vi "Remote Set Control Value.vi"(6 "Field name":string, 8 "error in (no error)":errorcluster, 10 "Name":string, 11 "Template Module in":refnum<class "Template Module.lvclass">) -> (0 "error out":errorcluster, 3 "Template Module out":refnum<class "Template Module.lvclass">, 9 "Value":variant)   [LabVIEW 2016]
uses:
  Template Module.lvclass
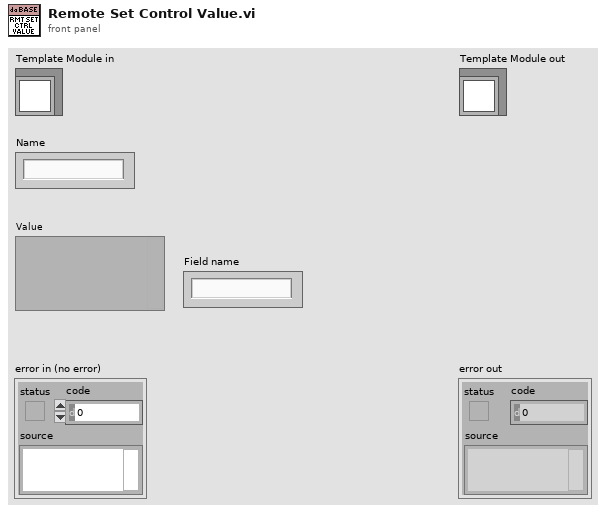
[diagram p1: front panel]
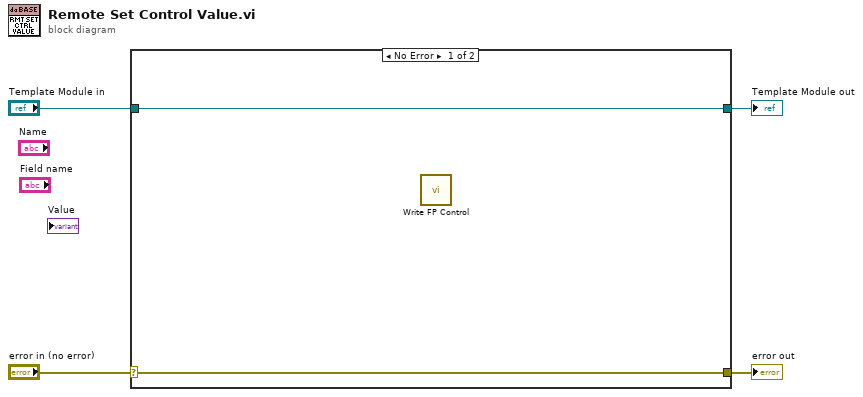
[diagram p0: block diagram]
diagram:
  n1 = case shown="No Error" "error in (no error)" {
    selector: "error in (no error)" -> [w5 w8]
    tunnel: [w5 w8] -> w3
    tunnel: [w6 w7] -> w1
    tunnel: "Template Module in" -> [w6 w7]
    frame No Error {
      n2 = call-dynamic "Write FP Control.vi"() -> ()  [unwired: 10 in, 2 out]
    }
    frame Error {
    }
  }
  "error out" <- w3
  "Template Module out" <- w1
